vi "varXNode_MessageWithoutEffect.vi"(0 "XRef":T5, 1 "Message In":T2, 2 "State In":T3) -> (14 "Message Out":T2, 15 "Reply":T1)   [LabVIEW 2017, in "varXNode.xnode"]
uses:
  <vilib>/variable/varXNode.llb/varXNode.xnode
  <vilib>/XNodeSupport/XNodeXNodeRef.ctl
  <vilib>/XNodeSupport/XNodeString.ctl
  <vilib>/variable/varXNode.llb/varXNode.ctl
  <vilib>/variable/Type Descriptor.ctl
  <vilib>/XNodeSupport/XNodeStringArray.ctl
  <vilib>/XNodeSupport/NI_XNodeSupport.lvlib
  <vilib>/variable/NI_Variable.lvlib
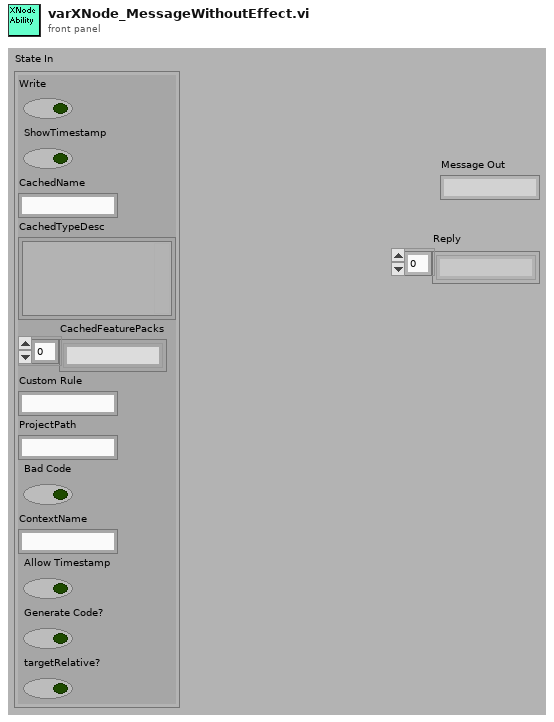
[diagram p1: front panel]
types:
  T1 = typedef "NI_XNodeSupport.lvlib/XNodeStringArray.ctl" = T2[]
  T2 = typedef "NI_XNodeSupport.lvlib/XNodeString.ctl" = string
  T3 = typedef "varXNode.xnode/varXNode.ctl" = cluster{"Write":bool, "ShowTimestamp":bool, "CachedName":string, "CachedTypeDesc":T4, "CachedFeaturePacks":string[], "Custom Rule":string, "ProjectPath":string, "Bad Code":bool, "ContextName":string, "Allow Timestamp":bool, "Generate Code?":bool, "targetRelative?":bool}
  T4 = typedef "NI_Variable.lvlib/Type Descriptor.ctl" = cluster{"Variant":variant}
  T5 = typedef "NI_XNodeSupport.lvlib/XNodeXNodeRef.ctl" = refnum<vi>
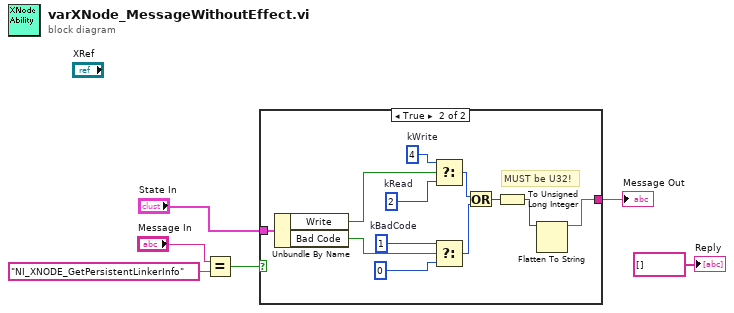
[diagram p0: block diagram]
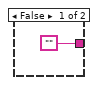
[diagram p2: hidden frame]
diagram:
  n1 = Equal?(x="Message In", y="NI_XNODE_GetPersistentLinkerInfo") -> (x = y?=w1:bool)
  n2 = case shown="True" w1 {
    tunnel: "State In" -> [_ w19]
    tunnel: ["" w9] -> w3
    frame False {
    }
    frame True {
      w15 = u32 1  # kBadCode
      w16 = u32 2  # kRead
      w17 = u32 4  # kWrite
      # "MUST be U32!"
      n3 = Unbundle By Name(w19) -> ("Write"=w18:bool, "Bad Code"=w13:bool)
      n4 = Select(t=w17, s=w18, f=w16) -> (s? t:f=w11:u32)
      n5 = Select(t=w15, s=w13, f=u32 0) -> (s? t:f=w12:u32)
      n6 = Or(x=w11, y=w12) -> (x .or. y?=w10:u32)
      n7 = To Unsigned Long Integer(number=w10) -> (unsigned 32bit integer=w8:u32)
      n8 = Flatten To String(anything=w8) -> (data string=w9:string)  [unwired: 3 in, 2 out]
    }
  }
  "Message Out" <- w3
  "Reply" <- T1 [] ("Reply")
